vi "main.vi"(0 "Tree":string(tree), 1 "Add":bool, 3 "Delete":bool, 11 "Error In":errorcluster, 12 "Save Data":bool, 13 "Load Data":bool, 14 "Combo Box":string(combo)="Add") -> (15 "Error Out":errorcluster)   [LabVIEW 2020]
doc: "This VI is to perform the math operations. Whereas the history of the operations will be saved in objects. \nThey can be retrived from the memory during the start of the VI."
uses:
  Typedef's/Q_Operations.ctl
  Typedef's/Data_Cluster.ctl
  Classes/Arithmetic_Operations/Arithmetic_Operations.lvclass
  Typedef's/UserEvent_Operations.ctl
  Typedef's/Event_Data.ctl
  Typedef's/Object_And_Name_Cluster.ctl
  <vilib>/Utility/error.llb/DialogType.ctl
  <vilib>/SLL Toolkit/SLL String/_SubVIs/I32 to String.vi
  <vilib>/Utility/xml.llb/Write to XML File(string).vi
  <vilib>/Utility/xml.llb/Read From XML File(string).vi
  <vilib>/SLL Toolkit/SLL String/SLL String.lvlib
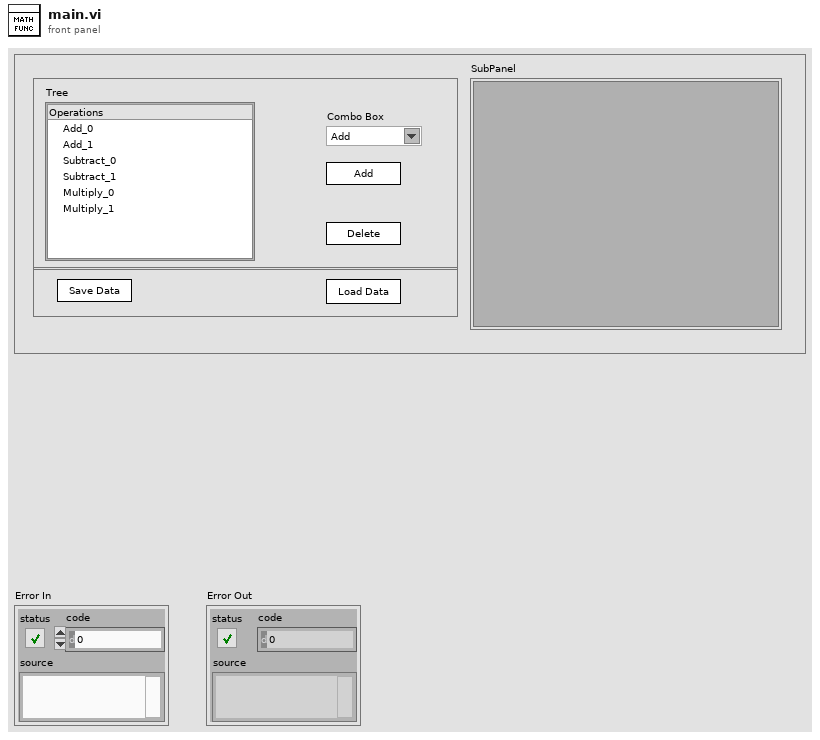
[diagram p1: front panel]
types:
  T1 = typedef "UserEvent_Operations.ctl" = enum16{"Create", "Generate", "Get Ref", "Destroy"}
  T2 = typedef "Data_Cluster.ctl" = cluster{"Operation Selected":string, "Objects Array":refnum<class "Arithmetic_Operations.lvclass">[], "Objects Count":cluster{"Add":i32, "Subtract":i32, "Multiply":i32, "Divide":i32}, "Prev Row Number":i32, "Num 1":dbl, "Num 2":dbl}
  T3 = typedef "Q_Operations.ctl" = enum16{"Create Q", "Enqueue", "Dequeue", "Enqueue N ele", "Enstack N ele", "Flush Q", "Destroy Q"}
  T4 = typedef "Event_Data.ctl" = cluster{"Stop Data":bool}
  T5 = typedef "Object_And_Name_Cluster.ctl" = cluster{"Object  Array":refnum<class "Arithmetic_Operations.lvclass">[], "Tree Entry":string[]}
  T6 = typedef "LVPoint32TypeDef.ctl" = cluster{"Horizontal":i32, "Vertical":i32}
  T7 = typedef "DialogType.ctl" = u16
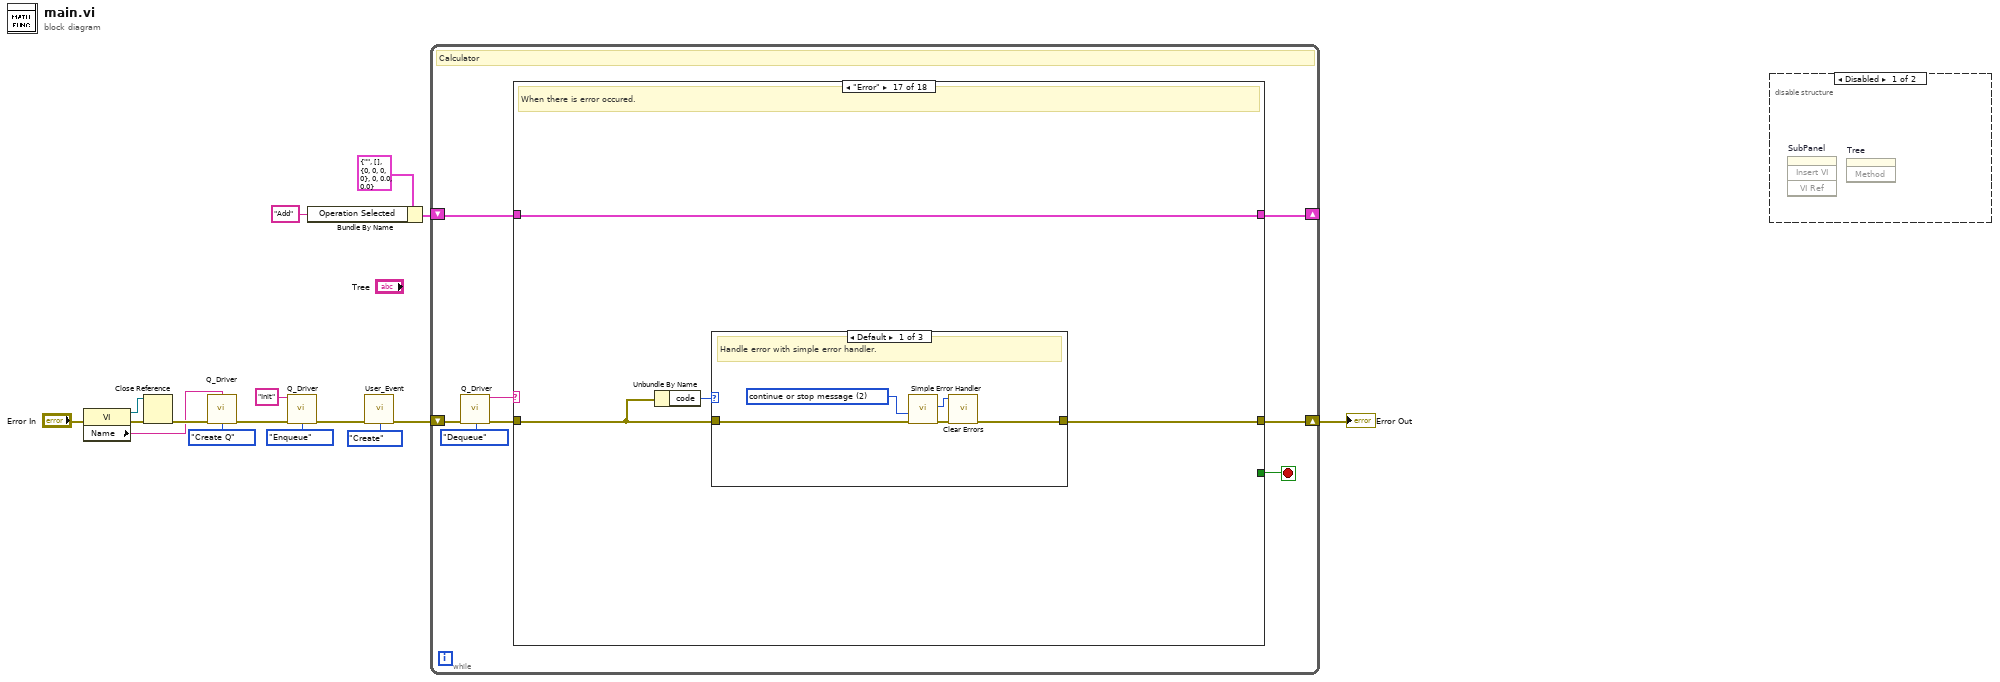
[diagram p0: block diagram]
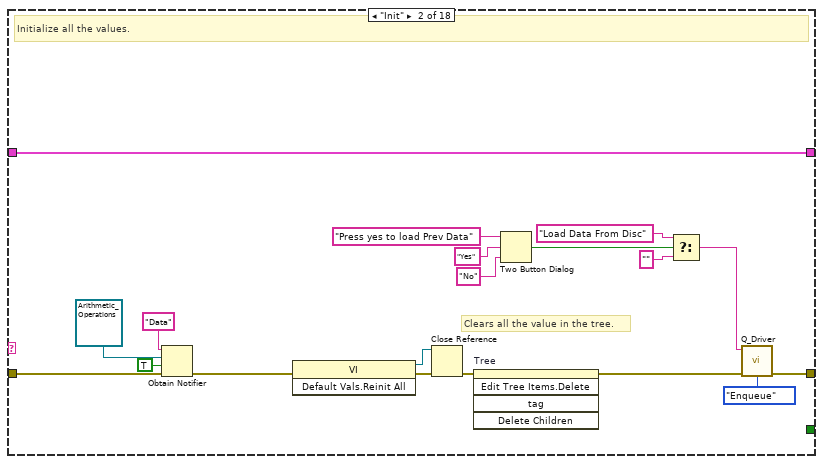
[diagram p4: hidden frame]
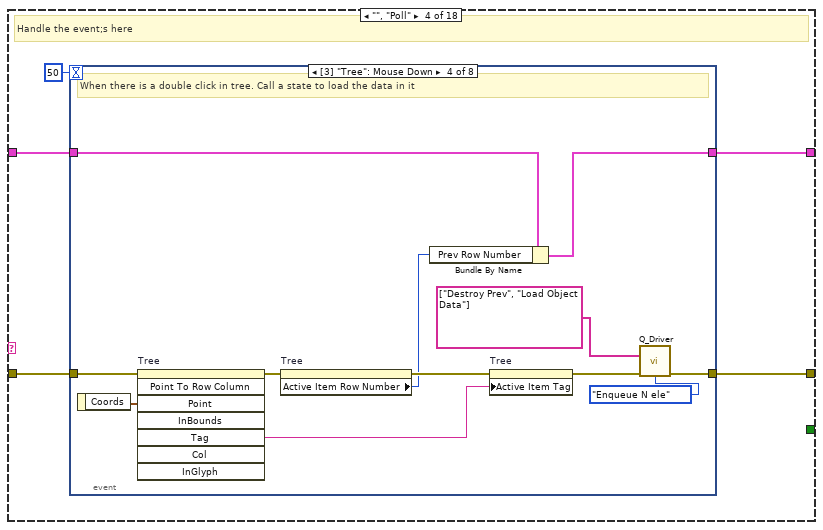
[diagram p6: hidden frame]
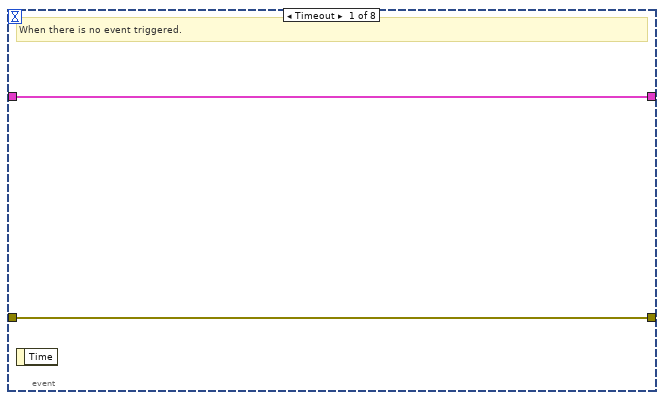
[diagram p7: hidden frame]
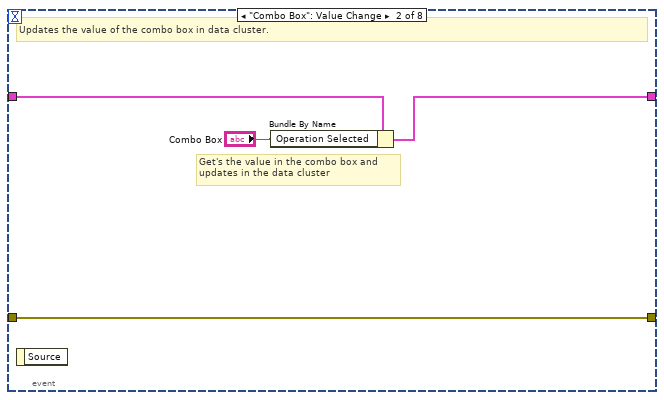
[diagram p8: hidden frame]
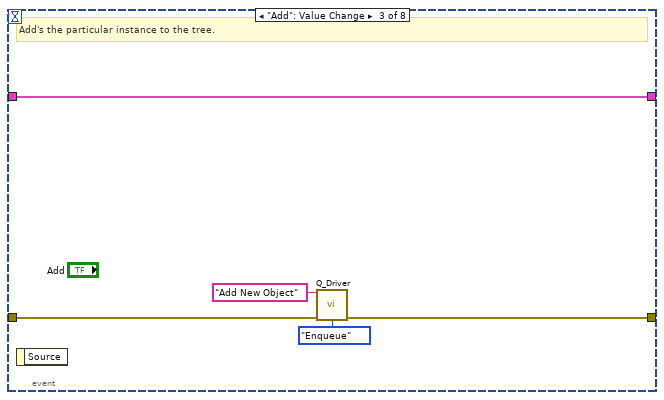
[diagram p9: hidden frame]
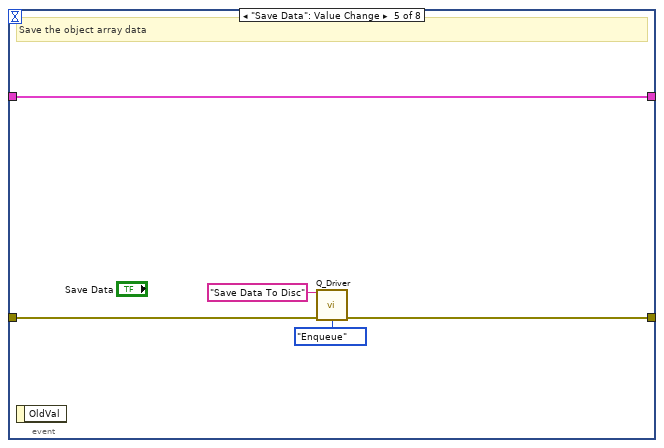
[diagram p10: hidden frame]
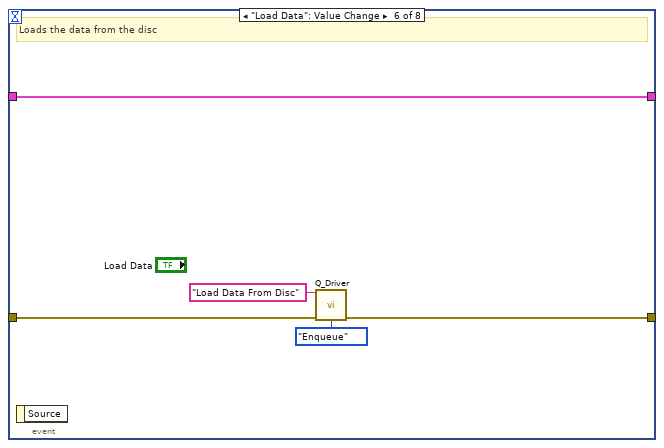
[diagram p11: hidden frame]
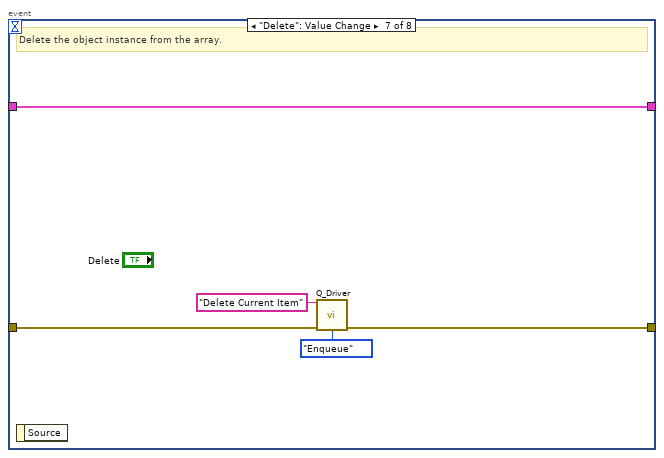
[diagram p12: hidden frame]
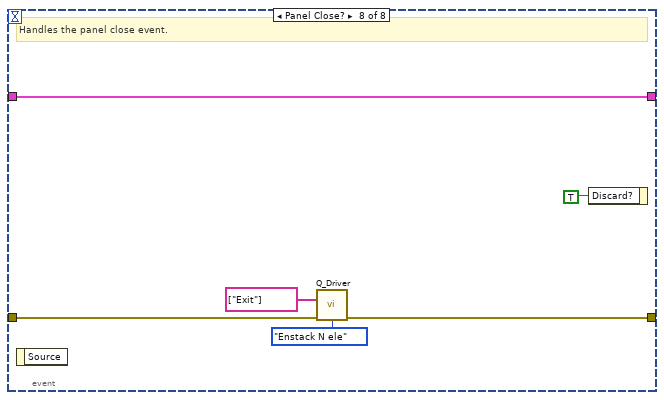
[diagram p13: hidden frame]
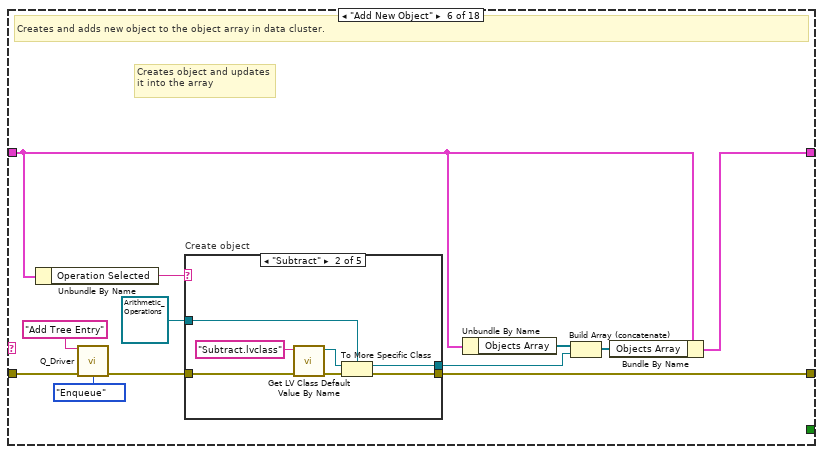
[diagram p15: hidden frame]
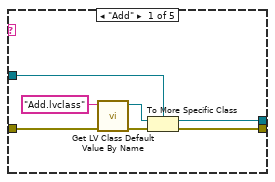
[diagram p16: hidden frame]
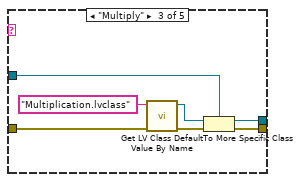
[diagram p17: hidden frame]
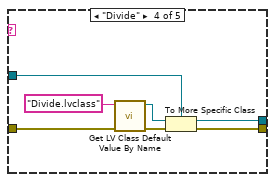
[diagram p18: hidden frame]
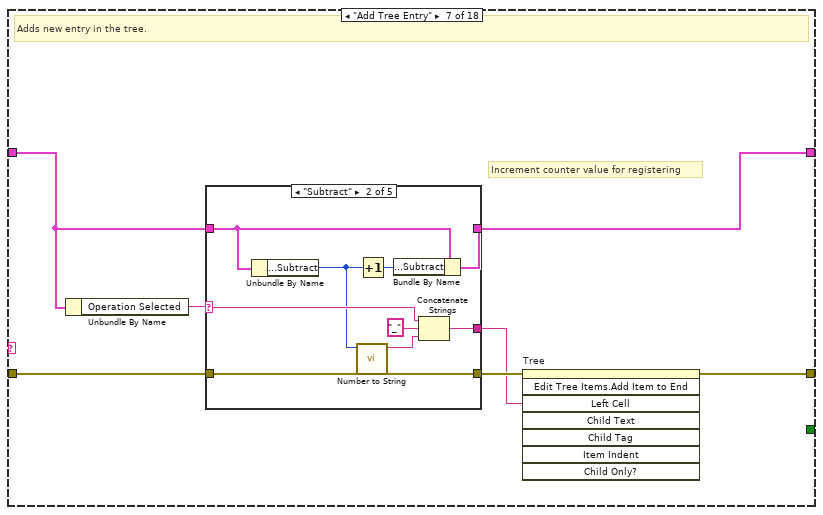
[diagram p20: hidden frame]
diagram:
  n1 = property class="VI"(error in="Error In") -> (reference out=w13:refnum<vi>, error out=w15:errorcluster, "Name"=w10:string)  [unwired: 1 in]
  n2 = Close Reference(reference=w13, error in (no error)=w15) -> (error out=w14:errorcluster)
  n3 = call "Q_Driver.vi"("Name"=w10, "Error In"=w14, "Operations"=Q_Operations."Create Q") -> ("Error Out"=w12:errorcluster)  [unwired: 11 in, 1 out]
  n4 = call "Q_Driver.vi"("State"="Init", "Error In"=w12, "Operations"=Q_Operations."Enqueue") -> ("Error Out"=w9:errorcluster)  [unwired: 11 in, 1 out]
  n5 = Bundle By Name(cluster=T2 {"Operation Selected"="", "Objects Array"=[], "Objects Count"={"Add"=0, "Subtract"=0, "Multiply"=0, "Divide"=0}, "Prev Row Number"=0, "Num 1"=0.0, "Num 2"=0.0} ("Data Cluster"), "Operation Selected"="Add") -> (w4:T2)
  n6 = call "User_Event.vi"("Error In"=w9, "Enum"=UserEvent_Operations."Create") -> ("Error Out"=w2:errorcluster)  [unwired: 12 in, 1 out]
  n7 = while {
    shift-right: [w20] -> w6
    shift-left: w2 -> [w23]
    shift-right: [w17] -> _
    shift-left: w4 -> [w18]
    stop <- w19 stop-if-true
    # "Calculator"
    n8 = call "Q_Driver.vi"("Error In"=w23, "Operations"=Q_Operations."Dequeue") -> ("Dequeued Element"=w21:string, "Error Out"=w24:errorcluster)  [unwired: 12 in]
    n9 = case shown="\"Error\"" w21 {
      tunnel: w24 -> [w26 w27 w47 w51 w98 w109 w144 w190 w216 w218 w228 w249 w257 w259 w260 w264 w266 w281]
      tunnel: [w26 w37 w47 w50 w98 w108 w143 w189 w214 w224 w229 w242 w257 w259 w260 w264 w267 w281] -> w20
      tunnel: [_ _ _ _ _ _ _ _ _ _ _ _ _ _ TRUE _ _ _] -> w19
      tunnel: w18 -> [w25 w38 w46 w49 w97 w106 w147 w186 w215 w225 w226 w247 w256 w258 w261 w263 w268 w280]
      tunnel: [w25 w38 w46 w48 w97 w103 w145 w187 w213 w225 w227 w243 w256 w258 w261 w263 w268 w280] -> w17
      frame "/**** Initialize ****/" {
      }
      frame "Init" {
        # "Clears all the value in the tree."
        # "Initialize all the values."
        n10 = Obtain Notifier(name (unnamed)="Data", notification data type=refnum<class "Arithmetic_Operations.lvclass"> refnum ("Arithmetic_Operations.lvclass"), create if not found? (T)=TRUE, error in (no error)=w27) -> (error out=w28:errorcluster)  [unwired: 2 out]
        n11 = invoke class="VI" method="Default Vals.Reinit All"(error in=w28) -> (reference out=w44:refnum<vi>, error out=w45:errorcluster)  [unwired: 2 in, 1 out]
        n12 = Close Reference(reference=w44, error in (no error)=w45) -> (error out=w43:errorcluster)
        n13 = invoke on="Tree" class="Tree (strict)" method="Edit Tree Items.Delete"(error in=w43) -> (error out=w39:errorcluster)  [unwired: 4 in, 4 out]
        n14 = Two Button Dialog(message="Press yes to load Prev Data", 1:"No" ("F button name (\"Cancel\")"), 2:"Yes" ("T button name (\"OK\")")) -> (T button?=w36:bool)
        n15 = Select(t="Load Data From Disc", s=w36, f="") -> (s? t:f=w33:string)
        n16 = call "Q_Driver.vi"("State"=w33, "Error In"=w39, "Operations"=Q_Operations."Enqueue") -> ("Error Out"=w37:errorcluster)  [unwired: 11 in, 1 out]
      }
      frame "/****Events*****/" {
      }
      frame "", "Poll" {
        # "Handle the event;s here"
        n17 = event shown="[3] \"Tree\": Mouse Down" {
          selector: _ -> [_ _ _ _ _ _ _ _]
          dyn-events: _ -> [_ _ _ _ _ _ _ _]
          timeout: 50 -> [_ _ _ _ _ _ _ _]
          tunnel: w51 -> [w54 w58 w63 w66 w80 w85 w90 w96]
          tunnel: [w54 w58 w61 w74 w78 w83 w88 w94] -> w50
          tunnel: [w53 w56 w62 w69 w79 w84 w89 w91] -> w48
          tunnel: w49 -> [w53 w57 w62 w75 w79 w84 w89 w91]
          event Timeout {
            # "When there is no event triggered."
            n18 = event-data() -> ()  [unwired: 1 in, 1 out]
          }
          event "Combo Box": Value Change {
            # "Get's the value in the combo box and\nupdates in the data cluster"
            # "Updates the value of the combo box in data cluster."
            n19 = event-data() -> ()  [unwired: 1 in, 1 out]
            n20 = Bundle By Name(cluster=w57, "Operation Selected"="Combo Box") -> (w56:T2)
          }
          event "Add": Value Change {
            # "Add's the particular instance to the tree."
            n21 = event-data() -> ()  [unwired: 1 in, 1 out]
            n22 = call "Q_Driver.vi"("State"="Add New Object", "Error In"=w63, "Operations"=Q_Operations."Enqueue") -> ("Error Out"=w61:errorcluster)  [unwired: 11 in, 1 out]
          }
          event "Tree": Mouse Down {
            # "When there is a double click in tree. Call a state to load the data in it"
            n23 = event-data() -> ("Coords"=w65:T6)  [unwired: 1 in]
            n24 = invoke on="Tree" class="Tree (strict)" method="Point To Row Column"(error in=w66, "Point"=w65) -> (error out=w67:errorcluster, "Tag"=w64:string)  [unwired: 6 in, 6 out]
            n25 = property on="Tree" class="Tree (strict)"(error in=w67) -> (error out=w70:errorcluster, "Active Item Row Number"=w68:i32)  [unwired: 1 in, 1 out]
            n26 = Bundle By Name(cluster=w75, "Prev Row Number"=w68) -> (w69:T2)
            n27 = property on="Tree" class="Tree (strict)"(error in=w70, "Active Item Tag"=w64) -> (error out=w72:errorcluster)  [unwired: 1 in, 1 out]
            n28 = call "Q_Driver.vi"("States[]"=string[] ["Destroy Prev", "Load Object Data"], "Error In"=w72, "Operations"=Q_Operations."Enqueue N ele") -> ("Error Out"=w74:errorcluster)  [unwired: 11 in, 1 out]
          }
          event "Save Data": Value Change {
            # "Save the object array data"
            n29 = event-data() -> ()  [unwired: 1 in, 1 out]
            n30 = call "Q_Driver.vi"("State"="Save Data To Disc", "Error In"=w80, "Operations"=Q_Operations."Enqueue") -> ("Error Out"=w78:errorcluster)  [unwired: 11 in, 1 out]
          }
          event "Load Data": Value Change {
            # "Loads the data from the disc"
            n31 = event-data() -> ()  [unwired: 1 in, 1 out]
            n32 = call "Q_Driver.vi"("State"="Load Data From Disc", "Error In"=w85, "Operations"=Q_Operations."Enqueue") -> ("Error Out"=w83:errorcluster)  [unwired: 11 in, 1 out]
          }
          event "Delete": Value Change {
            # "Delete the object instance from the array."
            n33 = event-data() -> ()  [unwired: 1 in, 1 out]
            n34 = call "Q_Driver.vi"("State"="Delete Current Item", "Error In"=w90, "Operations"=Q_Operations."Enqueue") -> ("Error Out"=w88:errorcluster)  [unwired: 11 in, 1 out]
          }
          event Panel Close? {
            # "Handles the panel close event."
            n35 = event-data() -> ()  [unwired: 1 in, 1 out]
            n36 = call "Q_Driver.vi"("States[]"=string[] ["Exit"], "Error In"=w96, "Operations"=Q_Operations."Enstack N ele") -> ("Error Out"=w94:errorcluster)  [unwired: 11 in, 1 out]
            n37 = event-data("Discard?"=TRUE) -> ()  [unwired: 1 in, 1 out]
          }
        }
      }
      frame "/**** Functionalities ***/" {
      }
      frame "Add New Object" {
        # "Creates object and updates it into the array"
        # "Creates and adds new object to the object array in data cluster."
        n38 = Unbundle By Name(w106) -> ("Operation Selected"=w110:string)
        n39 = call "Q_Driver.vi"("State"="Add Tree Entry", "Error In"=w109, "Operations"=Q_Operations."Enqueue") -> ("Error Out"=w101:errorcluster)  [unwired: 11 in, 1 out]
        n40 = case "Create object" shown="\"Subtract\"" w110 {
          tunnel: w101 -> [w115 w122 w129 w136 w140]
          tunnel: [w114 w121 w128 w135 w140] -> w108
          tunnel: refnum<class "Arithmetic_Operations.lvclass"> refnum ("Arithmetic_Operations.lvclass") -> [w112 w119 w126 w133 w139]
          tunnel: [w111 w118 w125 w132 w139] -> w104
          frame "Add" {
            # "Creates object for add"
            n41 = call <vilib>:"Get LV Class Default Value By Name.vi"("error in (no error)"=w115, "class name"="Add.lvclass") -> ("error out"=w116:errorcluster, "object"=w113:refnum<class>)  [unwired: 8 in]
            n42 = To More Specific Class(target class=w112, reference=w113, error in=w116) -> (specific class reference=w111:refnum<class "Arithmetic_Operations.lvclass">, error out=w114:errorcluster)
          }
          frame "Subtract" {
            n43 = call <vilib>:"Get LV Class Default Value By Name.vi"("error in (no error)"=w122, "class name"="Subtract.lvclass") -> ("error out"=w123:errorcluster, "object"=w120:refnum<class>)  [unwired: 8 in]
            n44 = To More Specific Class(target class=w119, reference=w120, error in=w123) -> (specific class reference=w118:refnum<class "Arithmetic_Operations.lvclass">, error out=w121:errorcluster)
          }
          frame "Multiply" {
            n45 = call <vilib>:"Get LV Class Default Value By Name.vi"("error in (no error)"=w129, "class name"="Multiplication.lvclass") -> ("error out"=w130:errorcluster, "object"=w127:refnum<class>)  [unwired: 8 in]
            n46 = To More Specific Class(target class=w126, reference=w127, error in=w130) -> (specific class reference=w125:refnum<class "Arithmetic_Operations.lvclass">, error out=w128:errorcluster)
          }
          frame "Divide" {
            n47 = call <vilib>:"Get LV Class Default Value By Name.vi"("error in (no error)"=w136, "class name"="Divide.lvclass") -> ("error out"=w137:errorcluster, "object"=w134:refnum<class>)  [unwired: 8 in]
            n48 = To More Specific Class(target class=w133, reference=w134, error in=w137) -> (specific class reference=w132:refnum<class "Arithmetic_Operations.lvclass">, error out=w135:errorcluster)
          }
          frame Default {
            # "When selection mismatches"
          }
        }
        n49 = Unbundle By Name(w106) -> ("Objects Array"=w105:refnum<class "Arithmetic_Operations.lvclass">[])
        n50 = Build Array (concatenate)(w105, w104) -> (w102:refnum<class "Arithmetic_Operations.lvclass">[])
        n51 = Bundle By Name(cluster=w106, "Objects Array"=w102) -> (w103:T2)
      }
      frame "Add Tree Entry" {
        # "Increment counter value for registering"
        # "Adds new entry in the tree."
        n52 = Unbundle By Name(w147) -> ("Operation Selected"=w146:string)
        n53 = case shown="\"Subtract\"" w146 {
          selector: w146 -> [w152 w159 w168 w176 _]
          tunnel: w147 -> [w156 w165 w174 w183 w185]
          tunnel: [w155 w164 w173 w182 w185] -> w145
          tunnel: w144 -> [w149 w160 w169 w178 w184]
          tunnel: [w149 w160 w169 w178 w184] -> w142
          tunnel: [w148 w157 w166 w175 _] -> w141
          frame "Add" {
            n54 = Unbundle By Name(w156) -> ("Objects Count.Add"=w153:i32)
            n55 = call-poly <vilib>:"Number to String.vi"("Numeric"=w153) -> ("String"=w151:string)  [unwired: 10 in]
            n56 = Increment(x=w153) -> (x+1=w154:i32)
            n57 = Bundle By Name(cluster=w156, "Objects Count.Add"=w154) -> (w155:T2)
            n58 = Concatenate Strings(w152, "_" ("string"), w151) -> (w148:string)
          }
          frame "Subtract" {
            n59 = Unbundle By Name(w165) -> ("Objects Count.Subtract"=w158:i32)
            n60 = call-poly <vilib>:"Number to String.vi"("Numeric"=w158) -> ("String"=w162:string)  [unwired: 10 in]
            n61 = Increment(x=w158) -> (x+1=w163:i32)
            n62 = Bundle By Name(cluster=w165, "Objects Count.Subtract"=w163) -> (w164:T2)
            n63 = Concatenate Strings(w159, "_" ("string"), w162) -> (w157:string)
          }
          frame "Multiply" {
            n64 = Unbundle By Name(w174) -> ("Objects Count.Multiply"=w167:i32)
            n65 = Increment(x=w167) -> (x+1=w172:i32)
            n66 = call-poly <vilib>:"Number to String.vi"("Numeric"=w167) -> ("String"=w171:string)  [unwired: 10 in]
            n67 = Bundle By Name(cluster=w174, "Objects Count.Multiply"=w172) -> (w173:T2)
            n68 = Concatenate Strings(w168, "_" ("string"), w171) -> (w166:string)
          }
          frame "Divide" {
            n69 = Unbundle By Name(w183) -> ("Objects Count.Divide"=w177:i32)
            n70 = call-poly <vilib>:"Number to String.vi"("Numeric"=w177) -> ("String"=w180:string)  [unwired: 10 in]
            n71 = Increment(x=w177) -> (x+1=w181:i32)
            n72 = Bundle By Name(cluster=w183, "Objects Count.Divide"=w181) -> (w182:T2)
            n73 = Concatenate Strings(w176, "_" ("string"), w180) -> (w175:string)
          }
          frame Default {
          }
        }
        n74 = invoke on="Tree" class="Tree (strict)" method="Edit Tree Items.Add Item to End"(error in=w142, "Left Cell"=w141) -> (error out=w143:errorcluster)  [unwired: 6 in, 7 out]
      }
      frame "Destroy Prev" {
        # "Destroy's the prev operation using the event."
        n75 = First Call?() -> (First Call?: T/F=w188:bool)
        n76 = case shown="False" w188 {
          tunnel: w190 -> [w203 w205]
          tunnel: [w196 w205] -> w189
          tunnel: w186 -> [w199 w204]
          tunnel: [w192 w204] -> w187
          frame False {
            # "After first call do these operation."
            n77 = invoke on="SubPanel" class="SubPnl" method="Remove VI"(error in=w203) -> (error out=w202:errorcluster)  [unwired: 2 in, 2 out]
            n78 = call "User_Event.vi"("Event Data"=T4 {"Stop Data"=TRUE}, "Error In"=w202, "Enum"=UserEvent_Operations."Generate") -> ("Error Out"=w197:errorcluster)  [unwired: 11 in, 1 out]
            n79 = Unbundle By Name(w199) -> ("Objects Array"=w195:refnum<class "Arithmetic_Operations.lvclass">[], "Prev Row Number"=w193:i32)
            n80 = Index Array(array=w195, index=w193) -> (element=w198:refnum<class "Arithmetic_Operations.lvclass">)
            n81 = call-dynamic "Get_Data.vi"("Arithmetic_Operations in"=w198, "Error In"=w197) -> ("Arithmetic_Operations out"=w194:refnum<class "Arithmetic_Operations.lvclass">, "Error Out"=w196:errorcluster)  [unwired: 12 in]
            n82 = Replace Array Subset(array=w195, new element=w194, index=w193) -> (w191:refnum<class "Arithmetic_Operations.lvclass">[])
            n83 = Bundle By Name(cluster=w199, "Objects Array"=w191) -> (w192:T2)
          }
          frame True {
            # "During first call do nothing."
          }
        }
      }
      frame "Load Object Data" {
        # "Loads the object data into the front panel."
        n84 = property on="Tree" class="Tree (strict)"(error in=w216) -> (error out=w206:errorcluster, "Active Item Row Number"=w211:i32)  [unwired: 1 in, 1 out]
        n85 = Unbundle By Name(w215) -> ("Objects Array"=w212:refnum<class "Arithmetic_Operations.lvclass">[])
        n86 = Index Array(array=w212, index=w211) -> (element=w208:refnum<class "Arithmetic_Operations.lvclass">)
        n87 = control-ref of="SubPanel"() -> (w207:refnum<vi>)
        n88 = call-dynamic "Talker.vi"("Arithmetic_Operations in"=w208, "Subpanel Ref"=w207, "Error In"=w206) -> ("Arithmetic_Operations out"=w209:refnum<class "Arithmetic_Operations.lvclass">, "Error Out"=w214:errorcluster)  [unwired: 11 in]
        n89 = Replace Array Subset(array=w212, new element=w209, index=w211) -> (w210:refnum<class "Arithmetic_Operations.lvclass">[])
        n90 = Bundle By Name(cluster=w215, "Objects Array"=w210) -> (w213:T2)
      }
      frame "Save Data To Disc" {
        # "Save's the object array data into the file system."
        n91 = property on="Tree" class="Tree (strict)"(error in=w218) -> (error out=w219:errorcluster, "All Tags"=w217:string[])  [unwired: 1 in, 1 out]
        n92 = Unbundle By Name(w225) -> ("Objects Array"=w221:refnum<class "Arithmetic_Operations.lvclass">[])
        n93 = Bundle By Name(cluster=T5 {"Object  Array"=[], "Tree Entry"=[]} ("Object and Name Array"), "Object  Array"=w221, "Tree Entry"=w217) -> (w220:T5)
        n94 = Flatten To XML(6:w220) -> (2:w223:string)
        n95 = call-poly <vilib>:"Write to XML File.vi"("error in (no error)"=w219, "XML Input"=w223) -> ("error out"=w224:errorcluster)  [unwired: 7 in, 2 out]
      }
      frame "Load Data From Disc" {
        # "Loads the data that is stored in the disc storage"
        n96 = call-poly <vilib>:"Read From XML File.vi"("error in (no error)"=w228) -> ("error out"=w236:errorcluster, "XML Elements"=w234:string)  [unwired: 8 in, 1 out]
        n97 = Unflatten From XML(xml string=w234, type=T5 {"Object  Array"=[], "Tree Entry"=[]} ("Object and Name Array"), error in (no error)=w236) -> (value=w233:T5, error out=w235:errorcluster)
        n98 = Unbundle By Name(w233) -> ("Object  Array"=w232:refnum<class "Arithmetic_Operations.lvclass">[], "Tree Entry"=w231:string[])
        n99 = Bundle By Name(cluster=w226, "Objects Array"=w232) -> (w227:T2)
        n100 = for {
          shift-right: [w238] -> w229
          shift-left: w235 -> [w239]
          tunnel: w231 -> [w237] mode=indexing
          # "Add all elements to tree"
          n101 = invoke on="Tree" class="Tree (strict)" method="Edit Tree Items.Add Item to End"(error in=w239, "Left Cell"=w237) -> (error out=w238:errorcluster)  [unwired: 6 in, 7 out]
        }
      }
      frame "Delete Current Item" {
        # "Deletes the current selected item from the table"
        n102 = property on="Tree" class="Tree (strict)"(error in=w249) -> (error out=w248:errorcluster, "Active Item Tag"=w241:string, "Active Item Row Number"=w245:i32)  [unwired: 1 in, 1 out]
        n103 = Unbundle By Name(w247) -> ("Objects Array"=w246:refnum<class "Arithmetic_Operations.lvclass">[])
        n104 = Delete From Array(array=w246, index=w245) -> (array with subset deleted=w244:refnum<class "Arithmetic_Operations.lvclass">[])  [unwired: 1 in, 1 out]
        n105 = Empty String/Path?(string/path=w241) -> (empty?=w240:bool)
        n106 = Bundle By Name(cluster=w247, "Objects Array"=w244) -> (w243:T2)
        n107 = case shown="False" w240 {
          tunnel: w248 -> [w253 w255]
          tunnel: [w250 w255] -> w242
          tunnel: w241 -> [w252 _]
          frame False {
            # "Destroy the current \noperation"
            # "When there is value in active tag"
            n108 = invoke on="Tree" class="Tree (strict)" method="Edit Tree Items.Delete"(error in=w253, "tag"=w252) -> (error out=w251:errorcluster)  [unwired: 3 in, 4 out]
            n109 = invoke on="SubPanel" class="SubPnl" method="Remove VI"(error in=w251) -> (error out=w250:errorcluster)  [unwired: 2 in, 2 out]
          }
          frame True {
            # "When there is no value in active tag"
            n110 = One Button Dialog(message="There is no Item selected. \nSelect any one item and press delete") -> ()  [unwired: 1 in, 1 out]
          }
        }
      }
      frame "/****Timer Operations*****/" {
      }
      frame "/***** Exit******/" {
      }
      frame "Exit" {
        # "Handles the exit state"
      }
      frame "/**** Error States ****/" {
      }
      frame "Error" {
        # "When there is error occured."
        n111 = Unbundle By Name(w266) -> ("code"=w265:i32)
        n112 = case shown="Default" w265 {
          selector: w265 -> [_ w274 w277]
          tunnel: [w272 w275 w278] -> w267
          tunnel: w266 -> [w269 w276 w279]
          frame Default {
            w270 = T7 2 items=["no dialog", "OK message", "continue or stop message", "OK message + warnings", "continue/stop + warnings"] ("type of dialog (OK msg:1)")
            # "Handle error with simple error handler."
            n113 = call <vilib>:"Simple Error Handler.vi"("type of dialog (OK msg:1)"=w270, "error in (no error)"=w269) -> ("code out"=w271:i32, "error out"=w273:errorcluster)  [unwired: 3 in, 3 out]
            n114 = call <vilib>:"Clear Errors.vi"("error in (no error)"=w273, "specific error code to clear (0: all)"=w271) -> ("error out"=w272:errorcluster)  [unwired: 4 in, 1 out]
          }
          frame 43 {
            n115 = call <vilib>:"Clear Errors.vi"("error in (no error)"=w276, "specific error code to clear (0: all)"=w274) -> ("error out"=w275:errorcluster)  [unwired: 4 in, 1 out]
          }
          frame 1136 {
            # "When no item is pressed in tree. (Clicked outside tree)"
            n116 = call <vilib>:"Clear Errors.vi"("error in (no error)"=w279, "specific error code to clear (0: all)"=w277) -> ("error out"=w278:errorcluster)  [unwired: 4 in, 1 out]
          }
        }
      }
      frame "Developer Error", Default {
        # "When there is any developer mistakes"
      }
    }
  }
  "Error Out" <- w6
  n117 = disable-structure shown="Disabled" {
    frame Disabled {
      n118 = invoke on="SubPanel" class="SubPnl" method="Insert VI"() -> ()  [unwired: 4 in, 4 out]
      n119 = invoke on="Tree" class="Tree (strict)" method=#-1() -> ()  [unwired: 3 in, 3 out]
    }
    frame Enabled {
    }
  }
